vi "EventCounterToEventCounterCluster.vi"(10 "EventCount":i32) -> (2 "CurrentRecordIndicator.EventCount":T1)   [LabVIEW 2020]
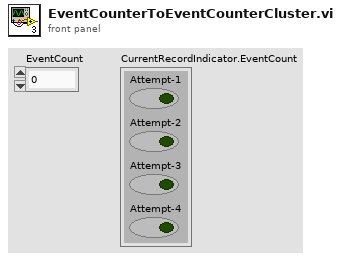
[diagram p1: front panel]
types:
  T1 = cluster{"Attempt-1":bool, "Attempt-2":bool, "Attempt-3":bool, "Attempt-4":bool}
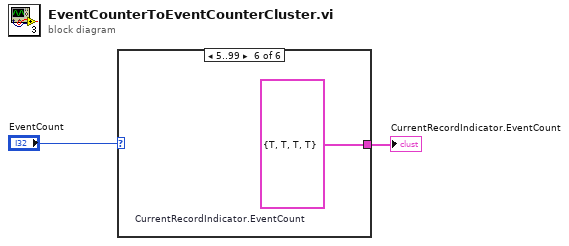
[diagram p0: block diagram]
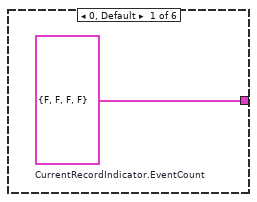
[diagram p2: hidden frame]
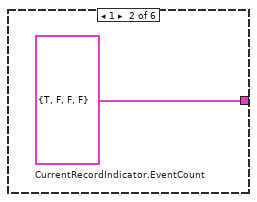
[diagram p3: hidden frame]
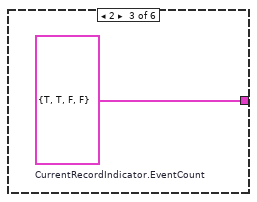
[diagram p4: hidden frame]
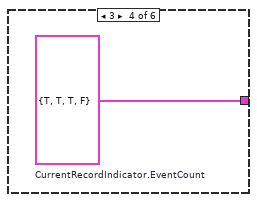
[diagram p5: hidden frame]
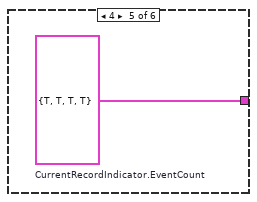
[diagram p6: hidden frame]
diagram:
  n1 = case shown="5..99" "EventCount" {
    tunnel: [w3 w4 w5 w6 w7 w8] -> w2
    frame 0, Default {
      w3 = T1 {"Attempt-1"=FALSE, "Attempt-2"=FALSE, "Attempt-3"=FALSE, "Attempt-4"=FALSE}  # CurrentRecordIndicator.EventCount
    }
    frame 1 {
      w4 = T1 {"Attempt-1"=TRUE, "Attempt-2"=FALSE, "Attempt-3"=FALSE, "Attempt-4"=FALSE}  # CurrentRecordIndicator.EventCount
    }
    frame 2 {
      w5 = T1 {"Attempt-1"=TRUE, "Attempt-2"=TRUE, "Attempt-3"=FALSE, "Attempt-4"=FALSE}  # CurrentRecordIndicator.EventCount
    }
    frame 3 {
      w6 = T1 {"Attempt-1"=TRUE, "Attempt-2"=TRUE, "Attempt-3"=TRUE, "Attempt-4"=FALSE}  # CurrentRecordIndicator.EventCount
    }
    frame 4 {
      w7 = T1 {"Attempt-1"=TRUE, "Attempt-2"=TRUE, "Attempt-3"=TRUE, "Attempt-4"=TRUE}  # CurrentRecordIndicator.EventCount
    }
    frame 5..99 {
      w8 = T1 {"Attempt-1"=TRUE, "Attempt-2"=TRUE, "Attempt-3"=TRUE, "Attempt-4"=TRUE}  # CurrentRecordIndicator.EventCount
    }
  }
  "CurrentRecordIndicator.EventCount" <- w2
